vi "testError.vi"() -> ()   [LabVIEW 2017, in "TestSuite.Tests.lvlib" / "Run.lvlib"]
uses:
  Run.lvlib
  TestSuite/TestSuite.lvclass
  Test/Test.lvclass
  Support/TestResultMock/TestResultMock.lvclass
  C:/Users/de200256/Code/logmanoriginal/lvunit/TestResult/TestResult.lvclass
  <vilib>/Utility/error.llb/Error Cluster From Error Code.vi
  <vilib>/ErrorRing/Error Ring.xnode
  Assertion/Assertion.lvlib
panel:
  out "error out":errorcluster
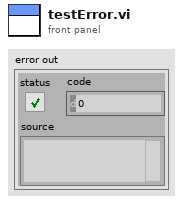
[diagram p1: front panel]
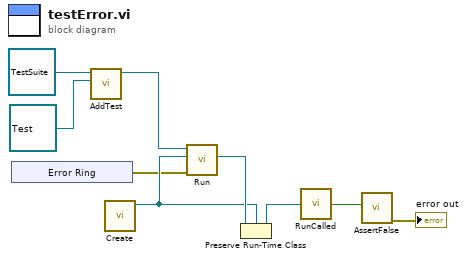
[diagram p0: block diagram]
diagram:
  n1 = xnode "Error Ring"() -> ("error out"=w4:errorcluster)
  n2 = call-dynamic "AddTest.vi"("Test"=refnum<class "Test.lvclass"> refnum ("TestCase"), "TestSuite in"=refnum<class "TestSuite.lvclass"> refnum ("TestSuite.lvclass")) -> ("TestSuite out"=w1:refnum<class "TestSuite.lvclass">)  [unwired: 8 in, 1 out]
  n3 = call "Create.vi"() -> ("TestResultMock"=w8:refnum<class "TestResultMock.lvclass">)  [unwired: 10 in, 1 out]
  n4 = call-dynamic "Run.vi"("error in (no error)"=w4, "TestResult"=w8, "TestSuite in"=w1) -> ("TestResult out"=w9:refnum<class "TestResult.lvclass">)  [unwired: 6 in, 2 out]
  n5 = Preserve Run-Time Class(object in=w9, 2:w8) -> (object out=w7:refnum<class "TestResultMock.lvclass">)  [unwired: 1 in, 1 out]
  n6 = call "RunCalled.vi"("TestResultMock In"=w7) -> ("Run Called"=w6:bool)
  n7 = call "AssertFalse.vi"("Condition"=w6) -> ("error out"=→"error out":errorcluster)  [unwired: 10 in]
